vi "vending_machine.vi"() -> ()   [LabVIEW 2018]
uses:
  TD_vending_machine_status.ctl
panel:
  out "Stato":T1
  in  "Annulla":bool
  out "messaggio":string
  out "somma":dbl
  out "resto":dbl
  in  "succo 0,60":bool
  in  "biscotti 1":bool
  in  "thè 0,35":bool
  in  "caffè 0,40":bool
  in  "#monete da 2":u8
  in  "#monete da 1":u8
  in  "#monete da 0,50":u8
  in  "#monete da 0,20":u8
  in  "#monete da 0,10":u8
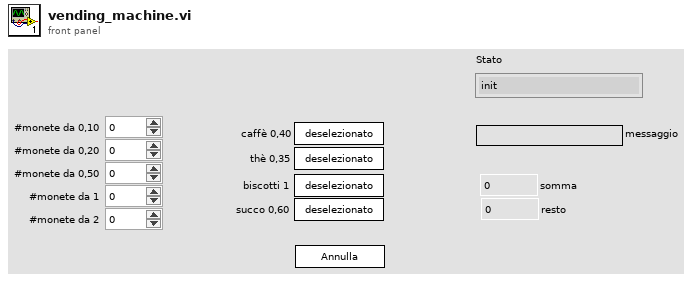
[diagram p1: front panel]
types:
  T1 = typedef "TD_vending_machine_status.ctl" = enum16{"init", "somma", "selezione", "valutazione", "uscita ok", "uscita notok"}
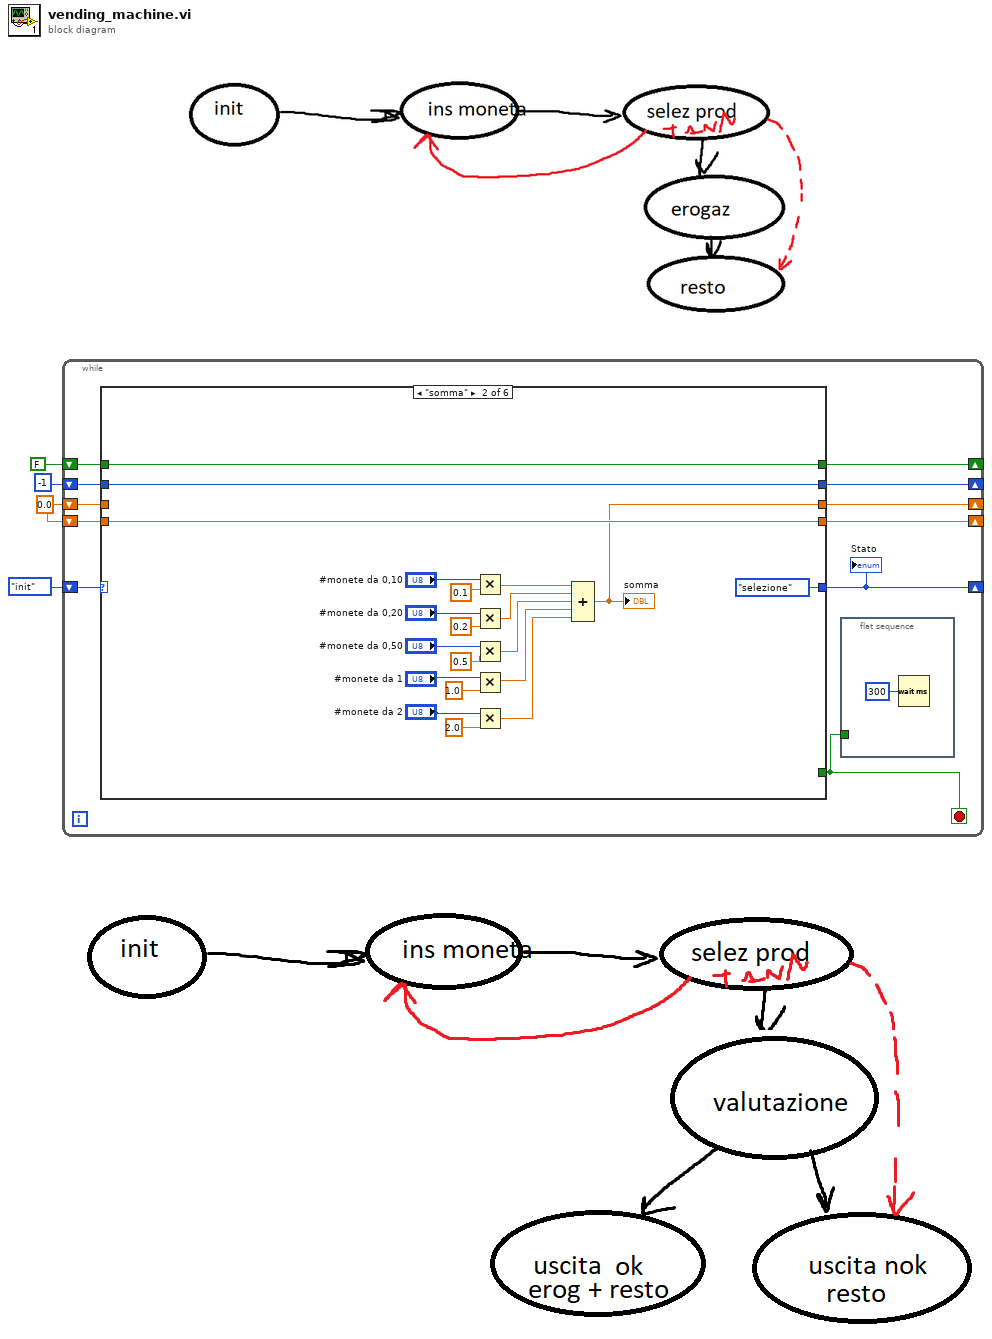
[diagram p0: block diagram]
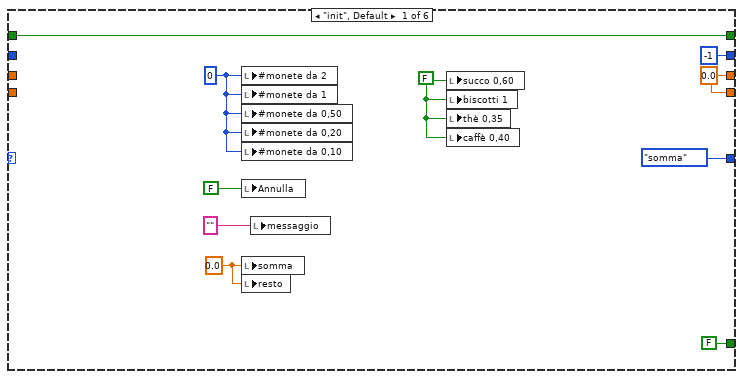
[diagram p2: hidden frame]
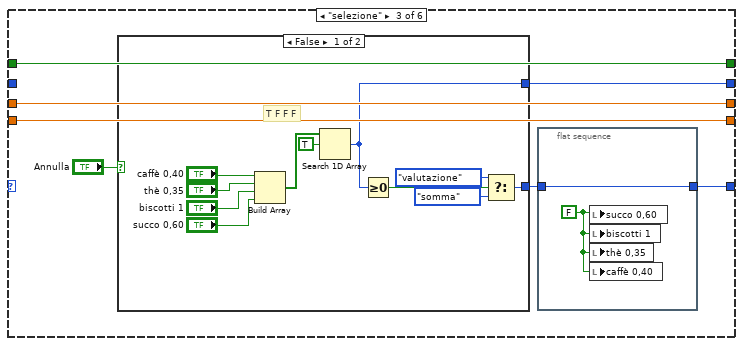
[diagram p3: hidden frame]
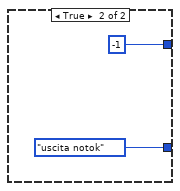
[diagram p4: hidden frame]
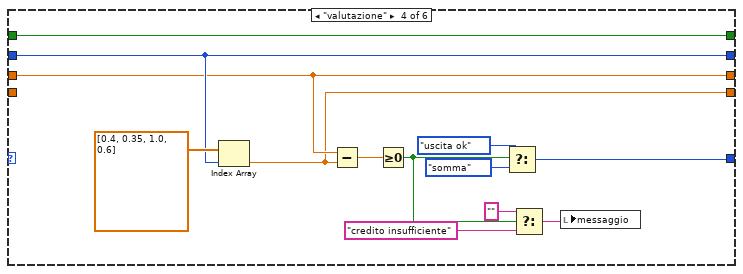
[diagram p5: hidden frame]
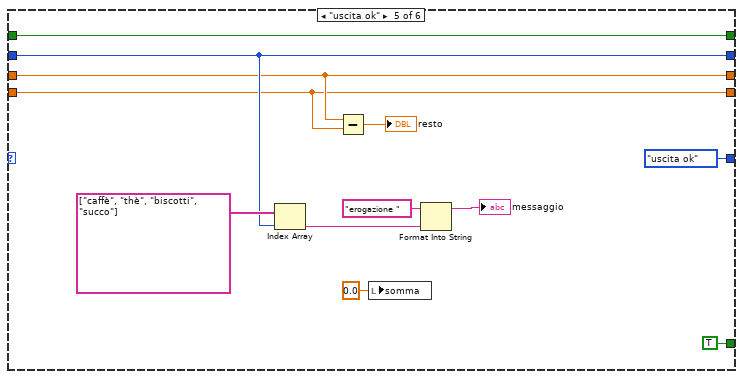
[diagram p6: hidden frame]
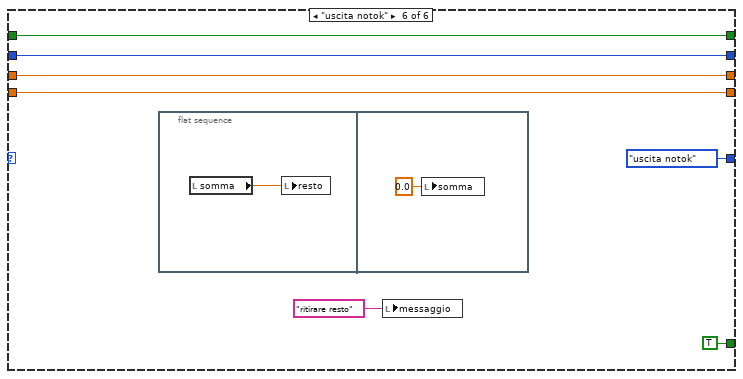
[diagram p7: hidden frame]
diagram:
  w2 = 0.0
  n1 = while {
    shift-right: [w13] -> _
    shift-left: FALSE -> [w14]
    shift-right: [w11] -> _
    shift-left: -1 ("index of element") -> [w12]
    shift-right: [w9] -> _
    shift-left: w2 -> [w10]
    shift-right: [w7] -> _
    shift-left: w2 -> [w8]
    shift-right: [w6] -> _
    shift-left: TD_vending_machine_status."init" ("Stato") -> [w15]
    stop <- w5 stop-if-true
    n2 = case shown="\"somma\"" w15 {
      tunnel: w14 -> [w26 w46 w53 w81 w93 w100]
      tunnel: [w26 w46 w53 w81 w93 w100] -> w13
      tunnel: w12 -> [_ w45 _ w79 w91 w99]
      tunnel: [-1 ("index of element") w45 w50 w79 w91 w99] -> w11
      tunnel: [w19 w42 w52 w78 w90 w98] -> w9
      tunnel: w10 -> [_ _ w52 w78 w90 w98]
      tunnel: w8 -> [_ w44 w51 _ w89 w97]
      tunnel: [w19 w44 w51 w74 w89 w97] -> w7
      tunnel: [FALSE _ _ _ TRUE TRUE] -> w5
      tunnel: [TD_vending_machine_status."somma" ("Stato") TD_vending_machine_status."selezione" ("Stato") w47 w75 TD_vending_machine_status."uscita ok" ("Stato") TD_vending_machine_status."uscita notok" ("Stato")] -> w6
      frame "init", Default {
        w17 = FALSE ("Annulla")
        w19 = 0.0
        w20 = 0.0 ("somma")
        w23 = u8 0 ("#monete da 2")
        n3 = local write "#monete da 2"(w23) -> ()
        n4 = local write "#monete da 1"(w23) -> ()
        n5 = local write "#monete da 0,50"(w23) -> ()
        n6 = local write "#monete da 0,20"(w23) -> ()
        n7 = local write "#monete da 0,10"(w23) -> ()
        n8 = local write "Annulla"(FALSE ("Annulla")) -> ()
        n9 = local write "somma"(w20) -> ()
        n10 = local write "resto"(w20) -> ()
        n11 = local write "messaggio"("" ("articolo scelto")) -> ()
        n12 = local write "succo 0,60"(w17) -> ()
        n13 = local write "biscotti 1"(w17) -> ()
        n14 = local write "thè 0,35"(w17) -> ()
        n15 = local write "caffè 0,40"(w17) -> ()
      }
      frame "somma" {
        n16 = Multiply(x="#monete da 0,10", y=0.1) -> (x*y=w41:dbl)
        n17 = Multiply(x="#monete da 0,20", y=0.2) -> (x*y=w30:dbl)
        n18 = Multiply(x="#monete da 0,50", y=0.5) -> (x*y=w29:dbl)
        n19 = Multiply(x="#monete da 1", y=1.0) -> (x*y=w28:dbl)
        n20 = Multiply(x="#monete da 2", y=2.0) -> (x*y=w27:dbl)
        n21 = Compound Arithmetic op=ADD(w41, w30, w29, w28, w27) -> (w42:dbl)
        "somma" <- w42
      }
      frame "selezione" {
        n22 = case shown="False" "Annulla" {
          tunnel: [w64 TD_vending_machine_status."uscita notok" ("f")] -> w48
          tunnel: [w57 -1 ("index of element")] -> w50
          frame False {
            # "T F F F"
            n23 = Build Array("caffè 0,40", "thè 0,35", "biscotti 1", "succo 0,60") -> (w59:bool[])
            n24 = Search 1D Array(1D array=w59, element=TRUE) -> (index of element=w57:i32)  [unwired: 1 in]
            n25 = Greater Or Equal To 0?(x=w57) -> (x >= 0?=w56:bool)
            n26 = Select(t=TD_vending_machine_status."valutazione" ("Stato"), s=w56, f=TD_vending_machine_status."somma") -> (s? t:f=w64:T1)
          }
          frame True {
          }
        }
        n27 = flat-sequence {
          tunnel: w48 -> [w55]
          tunnel: [w55] -> w47
          frame #0 {
            w54 = FALSE ("Annulla")
            n28 = local write "succo 0,60"(w54) -> ()
            n29 = local write "biscotti 1"(w54) -> ()
            n30 = local write "thè 0,35"(w54) -> ()
            n31 = local write "caffè 0,40"(w54) -> ()
          }
        }
      }
      frame "valutazione" {
        n32 = Index Array(array=dbl[] [0.4, 0.35, 1.0, 0.6], index=w79) -> (element=w74:dbl)
        n33 = Subtract(x=w78, y=w74) -> (x-y=w73:dbl)
        n34 = Greater Or Equal To 0?(x=w73) -> (x >= 0?=w72:bool)
        n35 = Select(t=TD_vending_machine_status."uscita ok" ("Stato"), s=w72, f=TD_vending_machine_status."somma" ("Stato")) -> (s? t:f=w75:T1)
        n36 = Select(t="", s=w72, f="credito insufficiente" ("messaggio")) -> (s? t:f=w71:string)
        n37 = local write "messaggio"(w71) -> ()
      }
      frame "uscita ok" {
        n38 = Index Array(array=string[] ["caffè", "thè", "biscotti", "succo"], index=w91) -> (element=w87:string)
        n39 = Subtract(x=w90, y=w89) -> (x-y=→"resto":dbl)
        n40 = local write "somma"(0.0 ("somma")) -> ()
        n41 = Format Into String(initial string="erogazione ", w87) -> (resulting string=→"messaggio":string)  [unwired: 2 in, 1 out]
      }
      frame "uscita notok" {
        n42 = flat-sequence {
          frame #0 {
            n43 = local read "somma"() -> (w101:dbl)
            n44 = local write "resto"(w101) -> ()
          }
          frame #1 {
            n45 = local write "somma"(0.0 ("somma")) -> ()
          }
        }
        n46 = local write "messaggio"("ritirare resto" ("articolo scelto")) -> ()
      }
    }
    "Stato" <- w6
    n47 = flat-sequence {
      tunnel: w5 -> [_]
      frame #0 {
        n48 = Wait (ms)(milliseconds to wait=u32 300) -> ()  [unwired: 1 out]
      }
    }
  }
